vi "Connection Wait.vi"(8 "error in":errorcluster, 10 "wait(ms)":u32=10000) -> (0 "error  out":errorcluster, 2 "Status Out":bool)   [LabVIEW 2022 SP3]
uses:
  Controls/All Loop Status.ctl
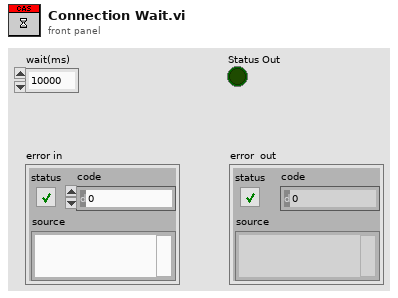
[diagram p1: front panel]
types:
  T1 = typedef "All Loop Status.ctl" = enum16{"AI", "AO", "DI", "DO", "TC", "Strain", "ACC", "RT", "Log"}
  T2 = enum16{"Init", "Read 'All'", "Read 'n'", "Read '1'", "Write '1'", "Write 'n'", "Write 'All'"}
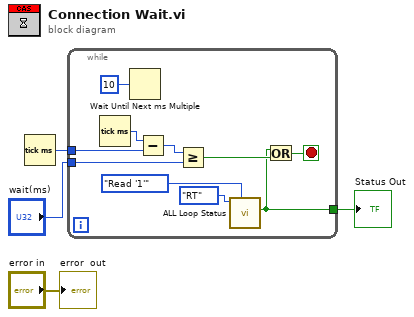
[diagram p0: block diagram]
diagram:
  n1 = Tick Count (ms)() -> (millisecond timer value=w4:u32)
  n2 = while {
    tunnel: w4 -> [w6]
    tunnel: "wait(ms)" -> [w9]
    tunnel: [w8] -> w1
    stop <- w10 stop-if-true
    n3 = Tick Count (ms)() -> (millisecond timer value=w7:u32)
    n4 = Wait Until Next ms Multiple(millisecond multiple=u32 10) -> ()  [unwired: 1 out]
    n5 = Subtract(x=w7, y=w6) -> (x-y=w14:u32)
    n6 = Greater Or Equal?(x=w14, y=w9) -> (x >= y?=w11:bool)
    n7 = call "ALL Loop Status.vi"("Option"=T2."Read '1'", "Loop"=All_Loop_Status."RT") -> ("Status Out"=w8:bool)  [unwired: 7 in, 2 out]
    n8 = Or(x=w8, y=w11) -> (x .or. y?=w10:bool)
  }
  "Status Out" <- w1
  "error  out" <- "error in"
